vi "New Stream To Disk Transport.vi"(9 "Channel Name":string, 10 "File Path":path) -> (0 "error out":errorcluster, 3 "StreamToDisk":refnum<class "StreamToDisk.lvclass">)   [LabVIEW 2015, in "Transport.lvlib" / "StreamToDisk.lvclass"]
doc: "<License>\nCopyright © 2017 Composed Systems, LLC | All rights reserved\nwww.composed.io\n\nAuthor: Ethan Stern <ethan.stern@composed.io>\n\nThis software is provided \"AS IS\" WITHOUT WARRANTIES, either express or implied, AND IS FOR EDUCATIONAL PURPOSES ONLY.\n</License>"
uses:
  StreamToDisk.lvclass
  StreamToDisk.lvclass/StreamToDisk.ctl
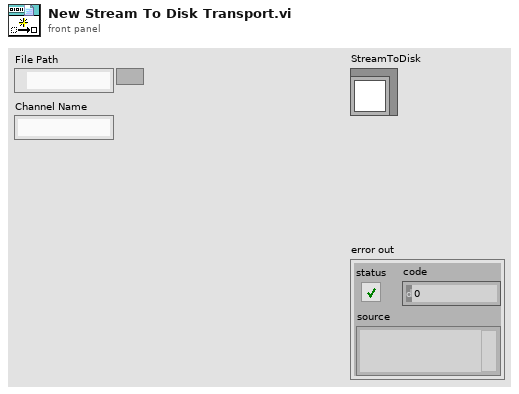
[diagram p1: front panel]
types:
  T1 = enum16{"open", "open or create", "create or replace", "create", "open (read-only)"}
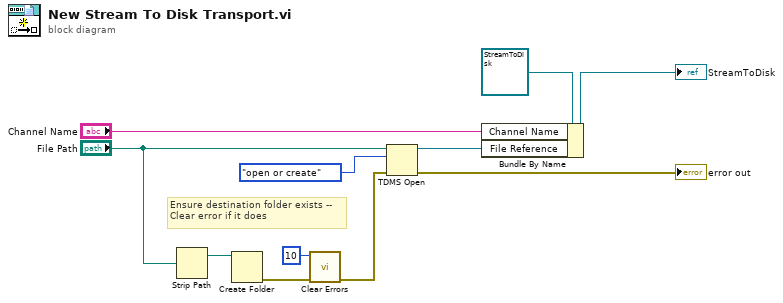
[diagram p0: block diagram]
diagram:
  # "Ensure destination folder exists --\nClear error if it does"
  n1 = Strip Path(path="File Path") -> (stripped path=w5:path)  [unwired: 1 out]
  n2 = Create Folder(path (use dialog)=w5) -> (error out=w4:errorcluster)  [unwired: 2 in, 2 out]
  n3 = call <vilib>:"Clear Errors.vi"("error in (no error)"=w4, "specific error code to clear (0: all)"=10) -> ("error out"=w2:errorcluster)  [unwired: 4 in, 1 out]
  n4 = TDMS Open(8:w2, 10:T1."open or create" ("operation (0:open)"), 11:"File Path") -> (0:→"error out":errorcluster, 3:w9:refnum<k34>)  [unwired: 4 in]
  n5 = Bundle By Name(cluster=refnum<class "StreamToDisk.lvclass"> refnum ("TerminalReference in"), "Channel Name"="Channel Name", "File Reference"=w9) -> (→"StreamToDisk":refnum<class "StreamToDisk.lvclass">)
